vi "Set Primary Destination Path.vi"(8 "error in (no error)":errorcluster, 10 "Destination path":path, 11 "Build in":refnum<class "NI_AB_API_SDIST.lvclass">) -> (0 "error out":errorcluster, 3 "Build out":refnum<class "NI_AB_API_SDIST.lvclass">)   [LabVIEW 2020, in "NI_AB_API_SDIST.lvclass"]
uses:
  <vilib>/AppBuilder/AB_API/SDIST/NI_AB_API_SDIST.lvclass
  <vilib>/AppBuilder/AB_API/SDIST/NI_AB_API_SDIST.lvclass/NI_AB_API_SDIST.ctl
  <vilib>/AppBuilder/AB_API/Build/NI_AB_API_Build.lvclass
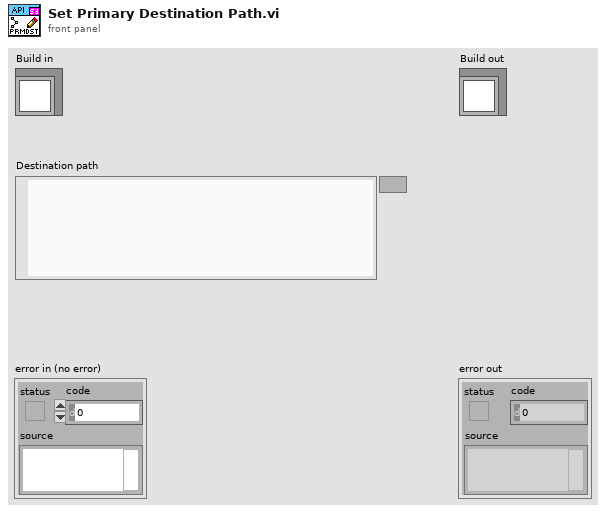
[diagram p1: front panel]
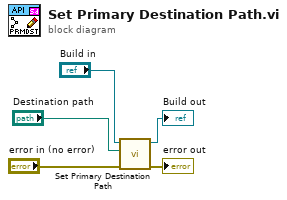
[diagram p0: block diagram]
diagram:
  n1 = call-parent "Set Primary Destination Path.vi"("error in (no error)"="error in (no error)", "Destination path"="Destination path", "Build in"="Build in") -> ("error out"=→"error out":errorcluster, "Build out"=→"Build out":refnum<class "NI_AB_API_SDIST.lvclass">)  [unwired: 7 in]
